vi "Save Window Location.vi"(4 "Error In":errorcluster, 7 "VI Refnum":refnum<vi>) -> (0 "Error Out":errorcluster, 3 "VI Refnum out":refnum<vi>)   [LabVIEW 2014, in "User Interface.lvlib"]
uses:
  User Interface.lvlib
  <vilib>/Utility/sysdir.llb/System Directory Type.ctl
  <vilib>/Utility/config.llb/Write Key (String).vi
  <vilib>/Utility/config.llb/NI_LVConfig.lvlib
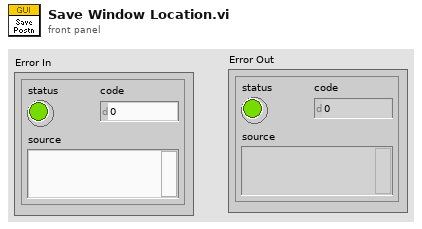
[diagram p1: front panel]
types:
  T1 = typedef "System Directory Type.ctl" = i32
  T2 = typedef "LVRectTypeDef.ctl" = cluster{"Left":i16, "Top":i16, "Right":i16, "Bottom":i16}
  T3 = typedef "NI_LVConfig.lvlib/Config Data RefNum.ctl" = refnum<k1>
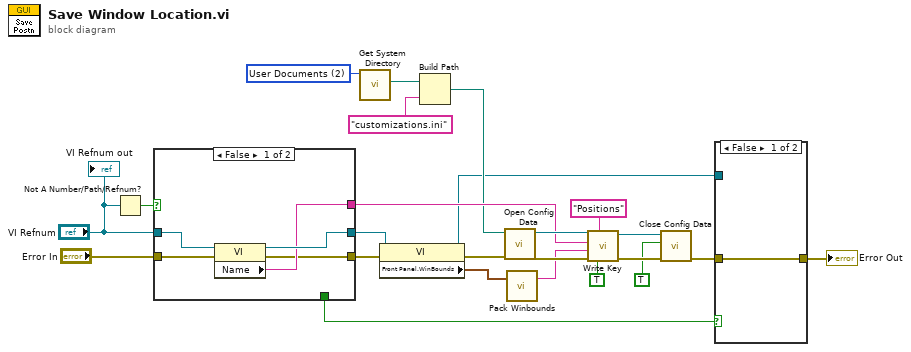
[diagram p0: block diagram]
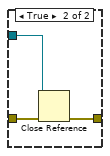
[diagram p2: hidden frame]
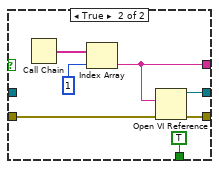
[diagram p3: hidden frame]
diagram:
  w10 = T1 2 items=["User Home"=0, "User Desktop"=1, "User Documents"=2, "User Application Data"=3, "User Preferences"=4, "User Temporary"=5, "Public Documents"=6, "Public Application Data"=7, "Public Preferences"=8, "Public Cache"=13, "System Core Libraries"=9, "System Installed Libraries"=10, "Application Files"=11, "Boot Volume Root"=12] ("system directory type")
  n1 = Not A Number/Path/Refnum?(number/path/refnum="VI Refnum") -> (NaN/Path/Refnum?=w15:bool)
  n2 = case shown="False" w15 {
    tunnel: [w26 w32] -> w12
    tunnel: "Error In" -> [w29 w34]
    tunnel: [w25 w33] -> w14
    tunnel: [w27 w31] -> w13
    tunnel: "VI Refnum" -> [w28 _]
    tunnel: [_ TRUE] -> w3
    frame False {
      n3 = property class="VI"(reference=w28, error in=w29) -> (reference out=w27:refnum<vi>, error out=w25:errorcluster, "Name"=w26:string)
    }
    frame True {
      n4 = Call Chain() -> (call chain=w36:string[])
      n5 = Index Array(array=w36, index=1) -> (element=w32:string)
      n6 = Open VI Reference(vi path=w32, error in (no error)=w34) -> (vi reference=w31:refnum<vi>, error out=w33:errorcluster)  [unwired: 4 in]
    }
  }
  n7 = call <vilib>:"Get System Directory.vi"("system directory type"=w10) -> ("system directory"=w9:path)  [unwired: 10 in]
  n8 = property class="VI"(reference=w13, error in=w14) -> (reference out=w1:refnum<vi>, error out=w2:errorcluster, "Front Panel.WinBounds"=w17:T2)
  n9 = Build Path(base path=w9, name or relative path="customizations.ini") -> (appended path=w8:path)
  n10 = call <vilib>:"Open Config Data.vi"("error in (no error)"=w2, "configuration file path"=w8) -> ("error out"=w24:errorcluster, "refnum"=w23:T3)  [unwired: 7 in, 1 out]
  n11 = call "Pack Winbounds.vi"("Front Panel.WinBounds"=w17) -> ("value"=w16:string)  [unwired: 2 in]
  n12 = call-poly <vilib>:"Write Key.vi"("write raw string? (F)"=TRUE ("read raw string? (F)"), "section"="Positions", "error in (no error)"=w24, "value"=w16, "key"=w12, "refnum"=w23) -> ("error out"=w21:errorcluster, "refnum out"=w20:T3)  [unwired: 3 in, 1 out]
  n13 = call <vilib>:"Close Config Data.vi"("error in (no error)"=w21, "write file if changed (T)"=TRUE ("read raw string? (F)"), "refnum"=w20) -> ("error out"=w4:errorcluster)  [unwired: 7 in, 1 out]
  n14 = case shown="False" w3 {
    tunnel: [w37 w38] -> w5
    tunnel: w4 -> [w37 w40]
    tunnel: w1 -> [_ w39]
    frame False {
    }
    frame True {
      n15 = Close Reference(reference=w39, error in (no error)=w40) -> (error out=w38:errorcluster)
    }
  }
  "Error Out" <- w5
  "VI Refnum out" <- "VI Refnum"
